vi "JSON TO VOLTAGE.vi"(7 "IP":string="192.168.23.100", 8 "error in (no error)":errorcluster, 10 "PORT":dbl=1.0 min=1.0 max=4.0 step=1.0, 11 "MASTER":dbl=1.0 min=1.0 max=10.0 step=1.0) -> (0 "error out":errorcluster, 3 "VOLTAGE":u32 format="%.0f V")   [LabVIEW 2024]
uses:
  <vilib>/JDP Science/JSONtext/JSONtext.lvlib
  <userlib>/_OpenG.lib/string/string.llb/openg_string.lvlib
panel:
  out "Response":string
  # "Smart connector voltage data"
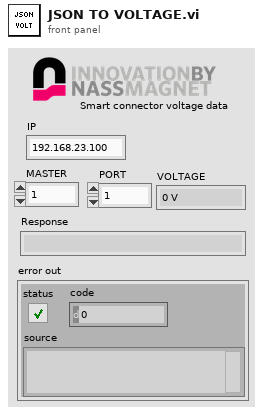
[diagram p1: front panel]
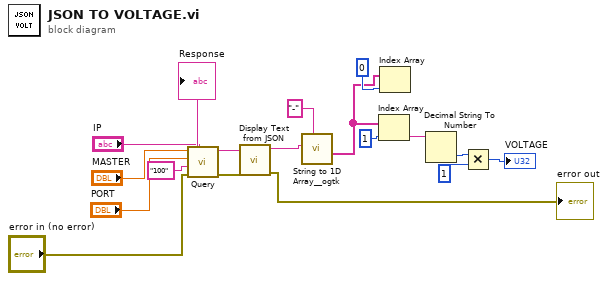
[diagram p0: block diagram]
diagram:
  n1 = call "Query.vi"("IP"="IP", "error in (no error)"="error in (no error)", "PARAMETERS"="100", "PORT"="PORT", "MASTER"="MASTER") -> ("error out"=w8:errorcluster, "JSON data"=w17:string)  [unwired: 5 in]
  "Response" <- w17
  n2 = call <vilib>:"Display Text from JSON.vi"("error in (no error)"=w8, "Input JSON"=w17) -> ("error out"=→"error out":errorcluster, "Display Text"=w5:string)  [unwired: 7 in, 1 out]
  n3 = call <userlib>:"String to 1D Array__ogtk.vi"("delimiter (Tab)"="-", "string"=w5) -> ("Array of Strings"=w12:string[])  [unwired: 9 in]
  n4 = Index Array(array=w12, index=1) -> (element=w6:string)
  n5 = Index Array(array=w12, index=0) -> ()  [unwired: 1 out]
  n6 = Decimal String To Number(string=w6) -> (number=w4:i32)  [unwired: 2 in, 1 out]
  n7 = Multiply(x=w4, y=u32 1) -> (x*y=→"VOLTAGE":u32)
